vi "parse extended err JSON.vi"(8 "error in (no error)":errorcluster, 11 "JSON string in":string) -> (0 "error out":errorcluster, 2 "jl error":bool, 3 "stack trace":T1)   [LabVIEW 2018, in "LV-0mq-Julia_roundtrip-lib.lvlib" / "LV2Julia_core.lvlib"]
uses:
  LV2Julia_core.lvlib
  detailed error info.ctl
  StackFrame.ctl
  extended error cluster.ctl
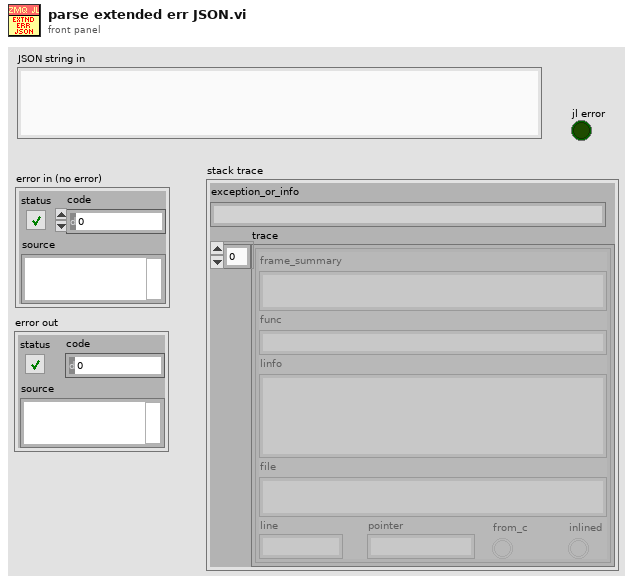
[diagram p1: front panel]
types:
  T1 = typedef "LV-0mq-Julia_roundtrip-lib.lvlib/LV2Julia_core.lvlib/detailed error info.ctl" = cluster{"exception_or_info":string, "trace":T2[]}
  T2 = typedef "LV-0mq-Julia_roundtrip-lib.lvlib/LV2Julia_core.lvlib/StackFrame.ctl" = cluster{"frame_summary":string, "func":string, "linfo":string, "file":string, "line":i32, "pointer":u64, "from_c":bool, "inlined":bool}
  T3 = typedef "LV-0mq-Julia_roundtrip-lib.lvlib/LV2Julia_core.lvlib/extended error cluster.ctl" = cluster{"errorinfo":cluster{"status":bool, "code":i32, "source":string, "detailed_info":T1}}
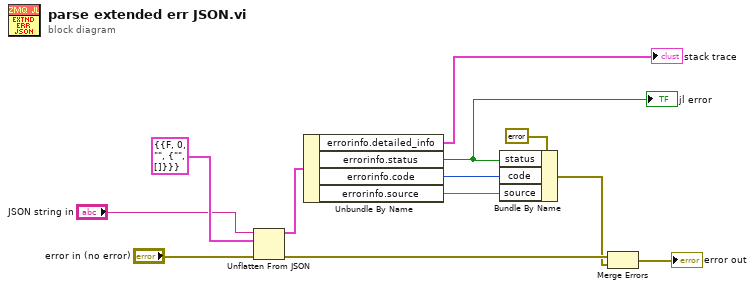
[diagram p0: block diagram]
diagram:
  n1 = Unflatten From JSON(JSON string="JSON string in", type and defaults=T3 {"errorinfo"={"status"=FALSE, "code"=0, "source"="", "detailed_info"={"exception_or_info"="", "trace"=[]}}} ("extended error"), error in (no error)="error in (no error)") -> (value=w12:T3, error out=w10:errorcluster)  [unwired: 4 in]
  n2 = Unbundle By Name(w12) -> ("errorinfo.detailed_info"=→"stack trace":T1, "errorinfo.status"=w4:bool, "errorinfo.code"=w5:i32, "errorinfo.source"=w6:string)
  "jl error" <- w4
  n3 = Bundle By Name(cluster=errorcluster {"status"=FALSE, "code"=0, "source"=""} ("input cluster"), "status"=w4, "code"=w5, "source"=w6) -> (w2:errorcluster)
  n4 = Merge Errors(w10, w2) -> (→"error out":errorcluster)
